vi "TargetOverride.vi"(0 "Override 1":bool=TRUE, 1 "Override 2":bool=TRUE caption="Override 1", 2 "Override 3":bool=TRUE caption="Override 1", 3 "Override 4":bool=TRUE caption="Override 1", 4 "Target set":i16[](array[ring]) items=["1", "2", "3", "4"]) -> (5 "Target set out":i16[](array[ring]) items=["1", "2", "3", "4"])   [LabVIEW 2010]
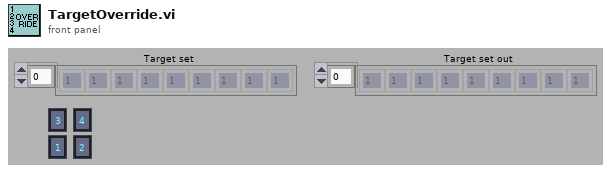
[diagram p1: front panel]
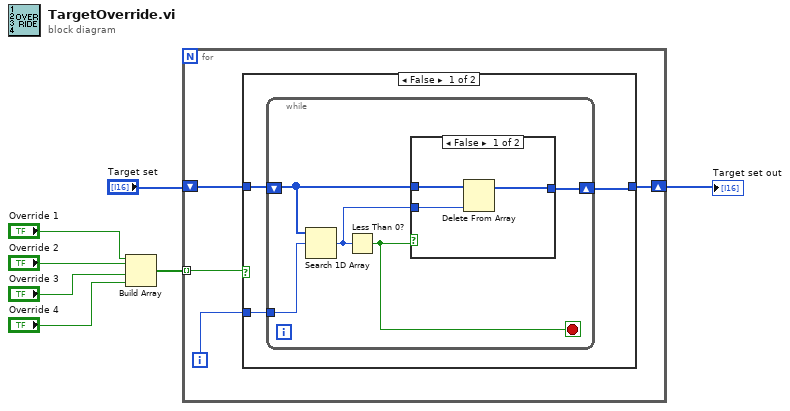
[diagram p0: block diagram]
diagram:
  n1 = Build Array("Override 1", "Override 2", "Override 3", "Override 4") -> (w3:bool[])
  n2 = for {
    tunnel: w3 -> [w11] mode=indexing
    shift-right: [w9] -> w1
    shift-left: "Target set" -> [w10]
    i -> [w8]
    n3 = case shown="False" w11 {
      tunnel: w10 -> [w13 w24]
      tunnel: [w12 w24] -> w9
      tunnel: w8 -> [w14 _]
      frame False {
        n4 = while {
          tunnel: w14 -> [w19]
          shift-right: [w16] -> w12
          shift-left: w13 -> [w17]
          stop <- w18 stop-if-true
          n5 = Search 1D Array(1D array=w17, element=w19) -> (index of element=w15:i32)  [unwired: 1 in]
          n6 = Less Than 0?(x=w15) -> (x < 0?=w18:bool)
          n7 = case shown="False" w18 {
            tunnel: w17 -> [w22 w23]
            tunnel: [w21 w23] -> w16
            tunnel: w15 -> [w20 _]
            frame False {
              n8 = Delete From Array(array=w22, index=w20) -> (array with subset deleted=w21:i16[])  [unwired: 1 in, 1 out]
            }
            frame True {
            }
          }
        }
      }
      frame True {
      }
    }
  }
  "Target set out" <- w1
